vi "AOL Z Cal-Optimal Motor Z start.vi"(7 "FOV info":cluster{"String":string, "Value":sgl}, 9 "FOVs":i32[](array[numeric]), 10 "Desired # cal points":i32, 11 "Current Cal (no Norm Z column)":dbl[][](array[numeric])) -> (3 "Optimal motor Z start positions":dbl[](array[numeric]))   [LabVIEW 2013]
uses:
  <vilib>/gmath/NI_Gmath.lvlib
panel:
  out "FOVs in current cal":i32
  out "Points in current cal":i32
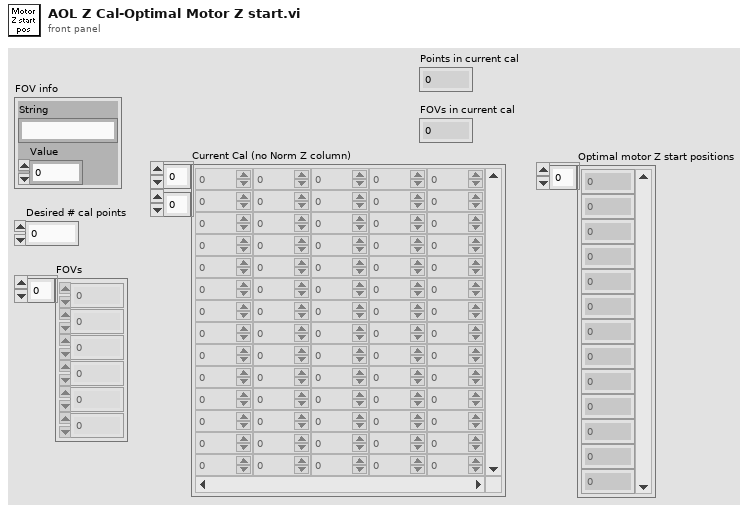
[diagram p1: front panel]
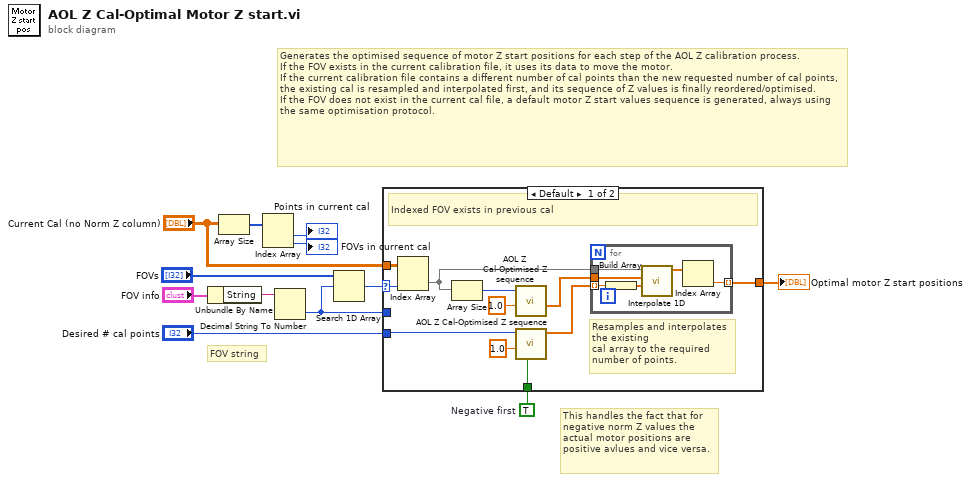
[diagram p0: block diagram]
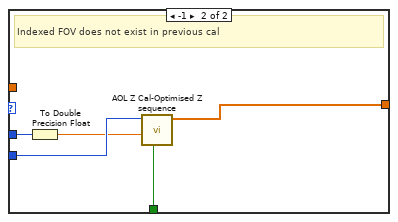
[diagram p2: hidden frame]
diagram:
  w1 = TRUE  # Negative first
  # "This handles the fact that for negative norm Z values the actual motor positions are positive avlues and vice versa."
  # "Generates the optimised sequence of motor Z start positions for each step of the AOL Z calibration process.\nIf the FOV exists in the current calibration file, it uses its data to move the motor.\nIf the current calibration file contains a different number of cal points than the new requested number of cal points, the existing cal is resampled and interpolated first, and its sequence of Z values is finally reordered/optimised.\nIf the FOV does not exist in the current cal file, a default motor Z start values sequence is generated, always using the same optimisation protocol."
  # "FOV string"
  n1 = Unbundle By Name("FOV info") -> ("String"=w11:string)
  n2 = Array Size(array="Current Cal (no Norm Z column)") -> (size(s)=w7:i32[])
  n3 = Index Array(array=w7) -> (element #1=→"Points in current cal":i32, element #2=→"FOVs in current cal":i32)  [unwired: 2 in]
  n4 = Decimal String To Number(string=w11) -> (number=w2:i32)  [unwired: 2 in, 1 out]
  n5 = Search 1D Array(1D array="FOVs", element=w2) -> (index of element=w9:i32)  [unwired: 1 in]
  n6 = case shown="Default" w9 {
    selector: w9 -> [w22 _]
    tunnel: "Desired # cal points" -> [w19 w34]
    tunnel: w2 -> [_ w33]
    tunnel: [w20 w32] -> w10
    tunnel: "Current Cal (no Norm Z column)" -> [w23 _]
    tunnel: w1 -> [w13 w30]
    frame Default {
      # "Resamples and interpolates the existing\ncal array to the required number of points."
      # "Indexed FOV exists in previous cal"
      n7 = Index Array(array=w23, index (col)=w22) -> (element=w21:dbl[])  [unwired: 1 in]
      n8 = Array Size(array=w21) -> (size(s)=w18:i32)
      n9 = call "AOL Z Cal-Optimised Z sequence.vi"("Max positive value"=1.0, "Calibration points"=w18) -> ("Decending order"=w16:dbl[])  [unwired: 8 in, 1 out]
      n10 = call "AOL Z Cal-Optimised Z sequence.vi"("Negative first (F)"=w13, "Max positive value"=1.0, "Calibration points"=w19) -> ("Calibration's optimised norm Z sequence"=w14:dbl[])  [unwired: 7 in, 1 out]
      n11 = for {
        tunnel: w14 -> [w28] mode=indexing
        tunnel: w16 -> [w25]
        tunnel: [w26] -> w20 mode=indexing
        tunnel: w21 -> [w24]
        n12 = Build Array(w28) -> (w27:dbl[])
        n13 = call <vilib>:"Interpolate 1D.vi"("xi"=w27, "X"=w25, "Y"=w24) -> ("yi"=w29:dbl[])  [unwired: 6 in, 2 out]
        n14 = Index Array(array=w29) -> (element=w26:dbl)  [unwired: 1 in]
      }
    }
    frame -1 {
      # "Indexed FOV does not exist in previous cal"
      n15 = To Double Precision Float(number=w33) -> (double precision float=w31:dbl)
      n16 = call "AOL Z Cal-Optimised Z sequence.vi"("Negative first (F)"=w30, "Max positive value"=w31, "Calibration points"=w34) -> ("Calibration's optimised norm Z sequence"=w32:dbl[])  [unwired: 7 in, 1 out]
    }
  }
  "Optimal motor Z start positions" <- w10
